vi "calculate dt.vi"(8 "f test":dbl, 9 "dt sampels":dbl, 10 "Array 2":cdb[](array[numeric]), 11 "Array":cdb[](array[numeric])) -> (3 "d t stream":dbl)   [LabVIEW 2021]
uses:
  <vilib>/Analysis/4window.llb/windowTd.ctl
  <vilib>/measure/NI_MAPro.lvlib
  <vilib>/Analysis/NI_AALPro.lvlib
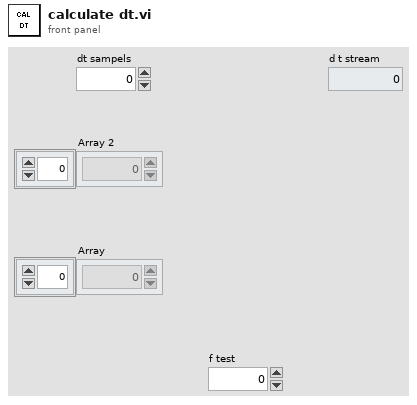
[diagram p1: front panel]
types:
  T1 = typedef "NI_AALPro.lvlib/windowTd.ctl" = u32
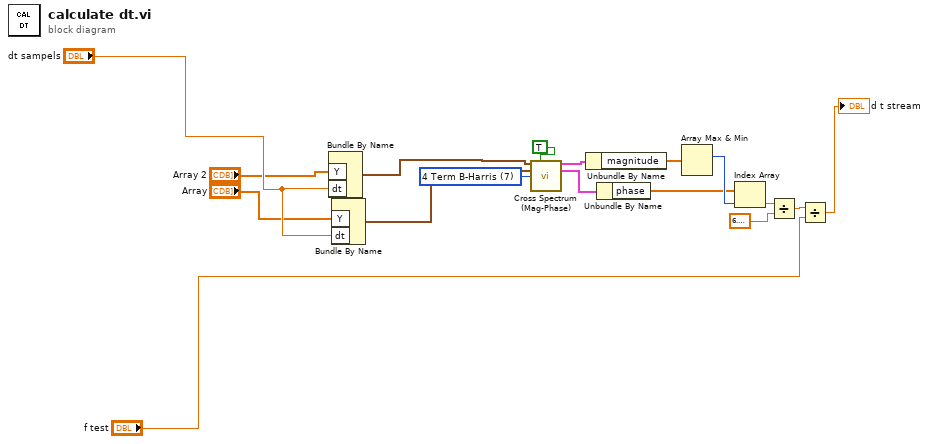
[diagram p0: block diagram]
diagram:
  w13 = T1 7 items=["Rectangle"=0, "Hanning"=1, "Hamming"=2, "Blackman-Harris"=3, "Exact Blackman"=4, "Blackman"=5, "Flat Top"=6, "4 Term B-Harris "=7, "7 Term B-Harris"=8, "Low Sidelobe"=9, "Blackman Nuttall"=11, "Triangle"=30, "Bartlett-Hanning"=31, "Bohman"=32, "Parzen"=33, "Welch"=34, "Kaiser"=60, "Dolph-Chebyshev"=61, "Gaussian"=62] ("window")
  n1 = Bundle By Name("Y"="Array 2", "dt"="dt sampels") -> (w14:waveform(cdb))  [unwired: 1 in]
  n2 = Bundle By Name("Y"="Array", "dt"="dt sampels") -> (w15:waveform(cdb))  [unwired: 1 in]
  n3 = call <vilib>:"Cross Spectrum (Mag-Phase).vi"("time signal X"=w14, "restart averaging (F)"=TRUE, "time signal Y"=w15, "window"=w13) -> ("magnitude"=w4:cluster{"f0":dbl, "df":dbl, "magnitude":dbl[]}, "phase"=w5:cluster{"f0":dbl, "df":dbl, "phase":dbl[]})  [unwired: 7 in, 3 out]
  n4 = Unbundle By Name(w4) -> ("magnitude"=w6:dbl[])
  n5 = Unbundle By Name(w5) -> ("phase"=w7:dbl[])
  n6 = Array Max & Min(array=w6) -> (max index (indices)=w8:i32)  [unwired: 3 out]
  n7 = Index Array(array=w7, index=w8) -> (element=w9:dbl)
  n8 = Divide(x=w9, y=6.283185307179586) -> (x/y=w10:dbl)
  n9 = Divide(x=w10, y="f test") -> (x/y=→"d t stream":dbl)
